vi "Xeryon process command.vi"(4 "Command in":string, 5 "Type":T1) -> (1 "Command out":string)   [LabVIEW 2014]
uses:
  Axis Manager/Axis enum.ctl
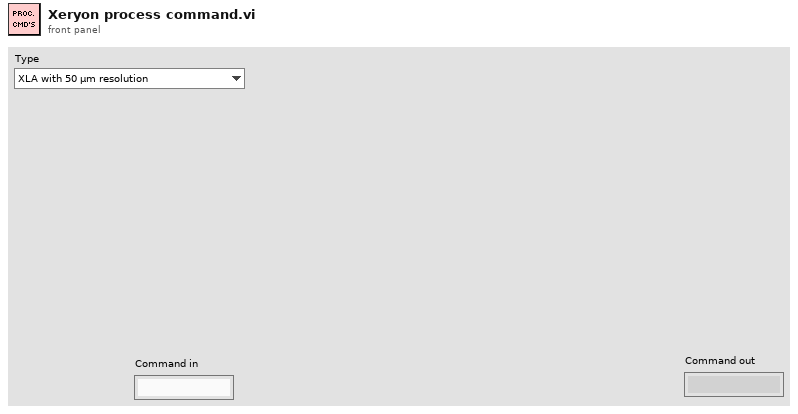
[diagram p1: front panel]
types:
  T1 = typedef "Axis enum.ctl" = enum16{"XLA with 50 µm resolution", "XLA with 10 µm resolution", "XLA with 1250 nm resolution", "XLA with 312 nm resolution", "XLA with 78 nm resolution", "XLS with 1250 nm resolution", "XLS with 312 nm resolution", "XLS with 78nm resolution", "XLS with 5nm resolution", "XLS with 1 nm resolution", "XRT-A with 109 µrad resolution", "XRT-U-30 with 109 µrad resolution", "XRT-U-30 with 49 µrad resolution", "XRT-U-30 with 19 µrad resolution", "XRT-U-30 with 3 µrad resolution", "XRT-U-40 with 109 µrad resolution", "XRT-U 40 with 49 µrad resolution", "XRT-U-40 with 19 µrad resolution", "XRT-U-40 with 3 µrad resolution", "XRT-U-60 with 109 µrad resolution", "XRT-U-60 with 49 µrad resolution", "XRT-U-60 with 19 µrad resolution", "XRT-U-60 with 3 µrad resolution"}
  T2 = enum16{"Position : From user units", "Position : To user units"}
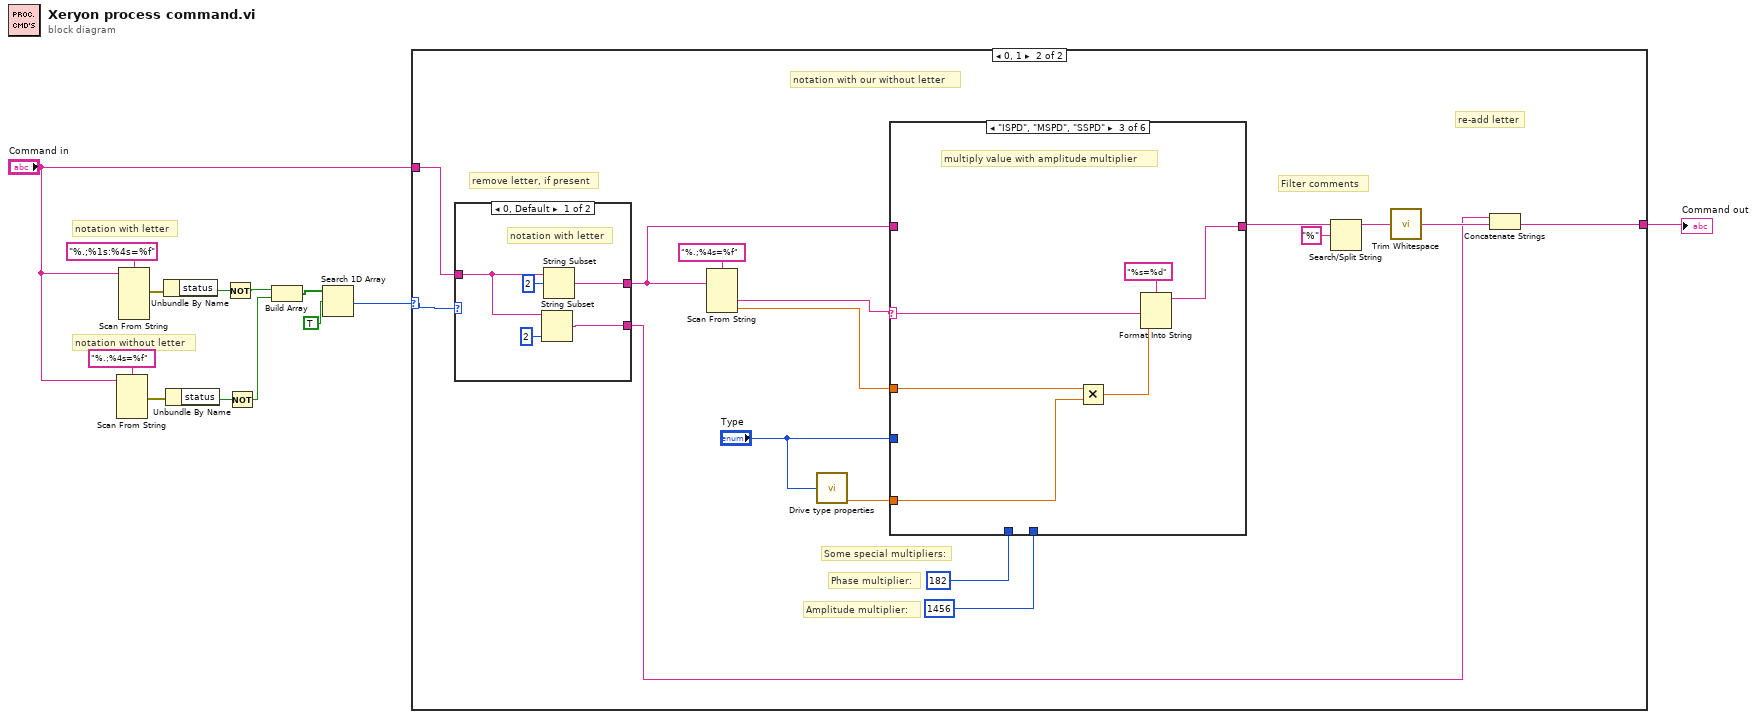
[diagram p0: block diagram]
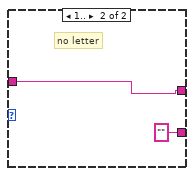
[diagram p3: hidden frame]
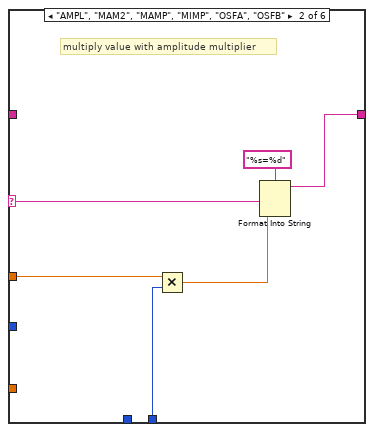
[diagram p5: hidden frame]
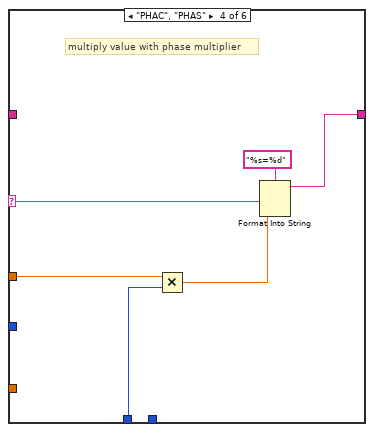
[diagram p6: hidden frame]
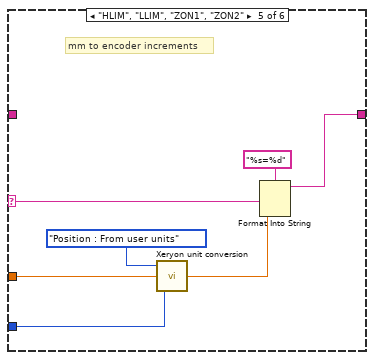
[diagram p7: hidden frame]
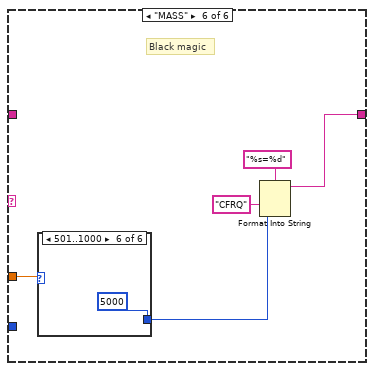
[diagram p8: hidden frame]
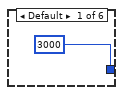
[diagram p9: hidden frame]
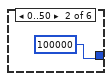
[diagram p10: hidden frame]
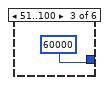
[diagram p11: hidden frame]
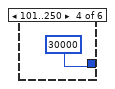
[diagram p12: hidden frame]
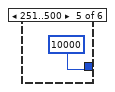
[diagram p13: hidden frame]
diagram:
  # "notation without letter"
  # "notation with letter"
  n1 = Scan From String(format string="%.;%4s=%f", input string="Command in") -> (error out=w7:errorcluster)  [unwired: 6 in, 2 out]
  n2 = Scan From String(format string="%.;%1s:%4s=%f", input string="Command in") -> (error out=w10:errorcluster)  [unwired: 8 in, 2 out]
  n3 = Unbundle By Name(w10) -> ("status"=w9:bool)
  n4 = Unbundle By Name(w7) -> ("status"=w8:bool)
  n5 = Not(x=w9) -> (.not. x?=w6:bool)
  n6 = Not(x=w8) -> (.not. x?=w5:bool)
  n7 = Build Array(w6, w5) -> (w4:bool[])
  n8 = Search 1D Array(1D array=w4, element=TRUE) -> (index of element=w2:i32)  [unwired: 1 in]
  n9 = case shown="0, 1" w2 {
    selector: w2 -> [_ w20]
    tunnel: [w14 w17] -> w12
    tunnel: "Command in" -> [w14 w25]
    frame -1, Default {
      # "don't change command"
      # "unknown notation"
    }
    frame 0, 1 {
      # "re-add letter"
      # "remove letter, if present"
      # "notation with our without letter"
      # "Filter comments"
      # "Phase multiplier:"
      # "Amplitude multiplier:"
      # "Some special multipliers:"
      n10 = case shown="0, Default" w20 {
        tunnel: w25 -> [w33 w37]
        tunnel: [w34 w37] -> w21
        tunnel: [w31 "" ("Command in")] -> w18
        frame 0, Default {
          # "notation with letter"
          n11 = String Subset(string=w33, length (rest)=2 ("length (rest)")) -> (substring=w31:string)  [unwired: 1 in]
          n12 = String Subset(string=w33, offset (0)=2) -> (substring=w34:string)  [unwired: 1 in]
        }
        frame 1.. {
          # "no letter"
        }
      }
      n13 = Scan From String(format string="%.;%4s=%f", input string=w21) -> (output 1=w23:string, output 2=w22:dbl)  [unwired: 4 in, 3 out]
      n14 = call "Drive type properties.vi"("Type"="Type") -> ("Speed multiplier"=w15:dbl)  [unwired: 2 in, 3 out]
      n15 = case shown="\"ISPD\", \"MSPD\", \"SSPD\"" w23 {
        selector: w23 -> [_ w41 w48 w54 w62 _]
        tunnel: [w38 w39 w46 w52 w61 w67] -> w28
        tunnel: w21 -> [w38 _ _ _ _ _]
        tunnel: w22 -> [_ w44 w50 w56 w59 w66]
        tunnel: 182 -> [_ _ _ w51 _ _]
        tunnel: 1456 -> [_ w43 _ _ _ _]
        tunnel: "Type" -> [_ _ _ _ w57 _]
        tunnel: w15 -> [_ _ w45 _ _ _]
        frame Default {
          # "Don't edit the command from the text file"
        }
        frame "AMPL", "MAM2", "MAMP", "MIMP", "OSFA", "OSFB" {
          # "multiply value with amplitude multiplier"
          n16 = Multiply(x=w44, y=w43) -> (x*y=w40:dbl)
          n17 = Format Into String(format string="%s=%d", w41, w40) -> (resulting string=w39:string)  [unwired: 2 in, 1 out]
        }
        frame "ISPD", "MSPD", "SSPD" {
          # "multiply value with amplitude multiplier"
          n18 = Multiply(x=w50, y=w45) -> (x*y=w47:dbl)
          n19 = Format Into String(format string="%s=%d", w48, w47) -> (resulting string=w46:string)  [unwired: 2 in, 1 out]
        }
        frame "PHAC", "PHAS" {
          # "multiply value with phase multiplier"
          n20 = Multiply(x=w56, y=w51) -> (x*y=w53:dbl)
          n21 = Format Into String(format string="%s=%d", w54, w53) -> (resulting string=w52:string)  [unwired: 2 in, 1 out]
        }
        frame "HLIM", "LLIM", "ZON1", "ZON2" {
          # "mm to encoder increments"
          n22 = call "Xeryon unit conversion.vi"("Type"=w57, "Value in"=w59, "Mode"=T2."Position : From user units") -> ("Value out"=w58:dbl)  [unwired: 2 in]
          n23 = Format Into String(format string="%s=%d", w62, w58) -> (resulting string=w61:string)  [unwired: 2 in, 1 out]
        }
        frame "MASS" {
          # "Black magic"
          n24 = case shown="501..1000" w66 {
            tunnel: [3000 100000 60000 30000 10000 5000] -> w64
            frame Default {
            }
            frame 0..50 {
            }
            frame 51..100 {
            }
            frame 101..250 {
            }
            frame 251..500 {
            }
            frame 501..1000 {
            }
          }
          n25 = Format Into String(format string="%s=%d", "CFRQ" ("input 1"), w64) -> (resulting string=w67:string)  [unwired: 2 in, 1 out]
        }
      }
      n26 = Search/Split String(string=w28, search string/char (-)="%") -> (substring before match=w26:string)  [unwired: 1 in, 2 out]
      n27 = call <vilib>:"Trim Whitespace.vi"("string"=w26) -> ("trimmed string"=w19:string)  [unwired: 1 in]
      n28 = Concatenate Strings(w18, w19) -> (w17:string)
    }
  }
  "Command out" <- w12
